vi "AutoDrawPaths.vi"(1 "RoutineName":string="untitled", 2 "Background File Path":path, 3 "RoutineSteps":T2[](array[typedef]) {"ArmPath"."ExtendTrajectory"."Time (ms)" items=["TrajectoryDuration_0ms"=0, "TrajectoryDuration_5ms"=5, "TrajectoryDuration_10ms"=10, "TrajectoryDuration_20ms"=20, "TrajectoryDuration_30ms"=30, "TrajectoryDuration_40ms"=40, "TrajectoryDuration_50ms"=50, "TrajectoryDuration_100ms"=100]; "ArmPath"."RotateTrajectory"."Time (ms)" items=["TrajectoryDuration_0ms"=0, "TrajectoryDuration_5ms"=5, "TrajectoryDuration_10ms"=10, "TrajectoryDuration_20ms"=20, "TrajectoryDuration_30ms"=30, "TrajectoryDuration_40ms"=40, "TrajectoryDuration_50ms"=50, "TrajectoryDuration_100ms"=100]}) -> ()   [LabVIEW 2018]
uses:
  TypeDef/AutoPreProcessedStep.ctl
  PathPlannerSupport/TypeDefs/DrivePlanResponse.ctl
  Pathfinder/Pathfinder-LabVIEW/Pathfinder-Lib/VIs/Segment.ctl
  Implements/Arm/TypeDefs/ArmPlanResponse.ctl
  General/MotionProfiling/TypeDefs/TrajectoryPoint.ctl
  <vilib>/Rock Robotics/WPI/ThirdParty/Phoenix-LabVIEW/Motor Controller/Controls/CTRE_Phoenix_MotorControl_TrajectoryPointTimeDur.ctl
  TypeDef/AutoWaypointType.ctl
  Implements/Arm/TypeDefs/ArmTargetPosition.ctl
  Implements/TypeDefs/IntakeState.ctl
  7e158850-ddb7-454d-ad08-8f74a83b50bd.vi
  ArgosLib/ArgosLib.lvlib
  Pathfinder/Pathfinder-LabVIEW/Pathfinder-Lib/Pathfinder.lvlib
panel:
  in  "Scale Factor":u8=2
  out "Image Out":T1(plugin-control)
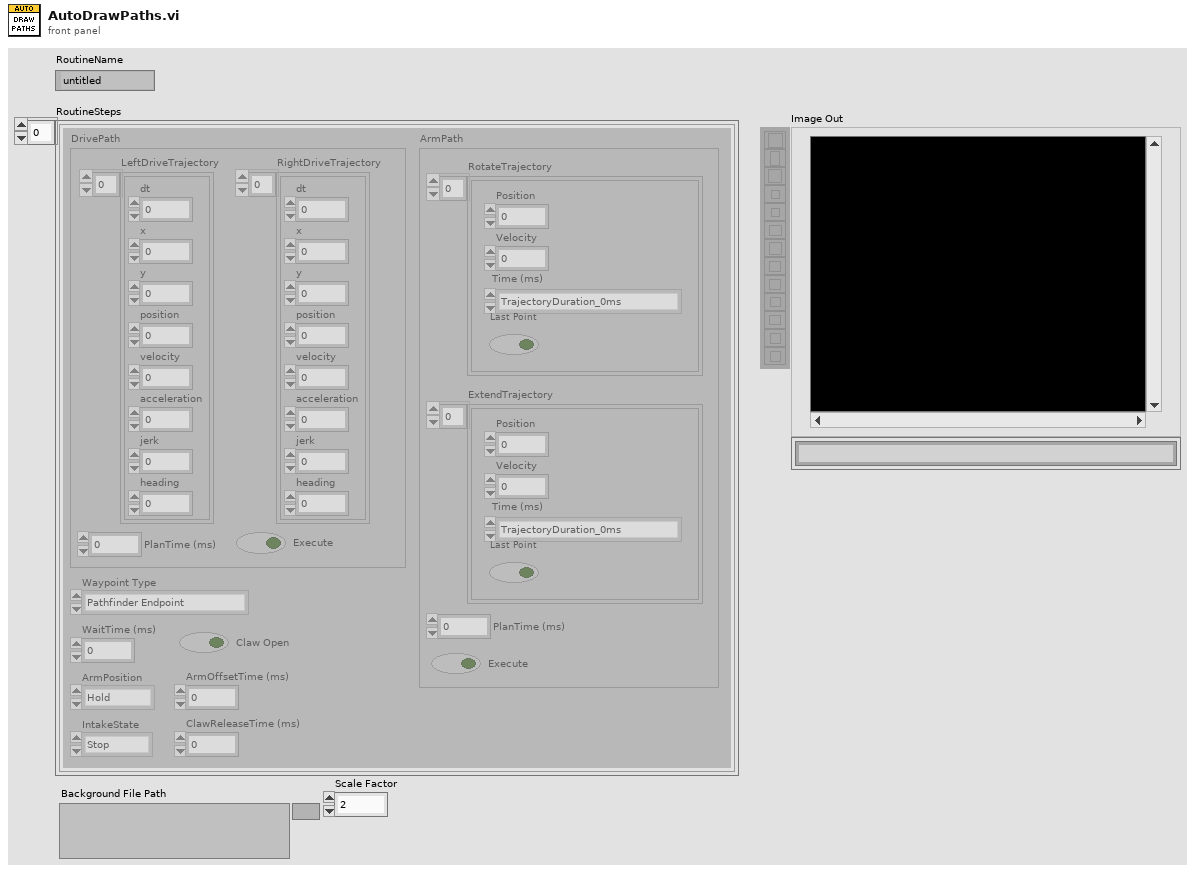
[diagram p1: front panel]
types:
  T1 = typedef "IMAQ Image.ctl" = refnum<image>
  T2 = typedef "AutoPreProcessedStep.ctl" = cluster{"DrivePath":T3, "ArmPath":T5, "Waypoint Type":T8, "WaitTime (ms)":u16, "ArmPosition":T9, "IntakeState":T10, "Claw Open":bool, "ArmOffsetTime (ms)":u16, "ClawReleaseTime (ms)":i32}
  T3 = typedef "DrivePlanResponse.ctl" = cluster{"LeftDriveTrajectory":T4[], "RightDriveTrajectory":T4[], "PlanTime (ms)":u32, "Execute":bool}
  T4 = typedef "Pathfinder.lvlib/Segment.ctl" = cluster{"dt":dbl, "x":dbl, "y":dbl, "position":dbl, "velocity":dbl, "acceleration":dbl, "jerk":dbl, "heading":dbl}
  T5 = typedef "ArmPlanResponse.ctl" = cluster{"RotateTrajectory":T6[], "ExtendTrajectory":T6[], "PlanTime (ms)":u32, "Execute":bool}
  T6 = typedef "TrajectoryPoint.ctl" = cluster{"Position ":dbl, "Velocity ":dbl, "Time (ms)":T7, "Last Point":bool}
  T7 = typedef "CTRE_Phoenix_MotorControl_TrajectoryPointTimeDur.ctl" = i32
  T8 = typedef "AutoWaypointType.ctl" = enum16{"Pathfinder Endpoint", "Pathfinder Waypoint", "Zero-Radius Turn Endpoint", "Stationary", "Vision Assist Endpoint", "Stop"}
  T9 = typedef "ArmTargetPosition.ctl" = enum16{"Hold", "Switch", "Scale Low", "Scale High", "Climb", "Back Place"}
  T10 = typedef "IntakeState.ctl" = enum16{"Stop", "Forward", "Reverse", "Forward Open"}
  T11 = typedef "Image Type" = u32
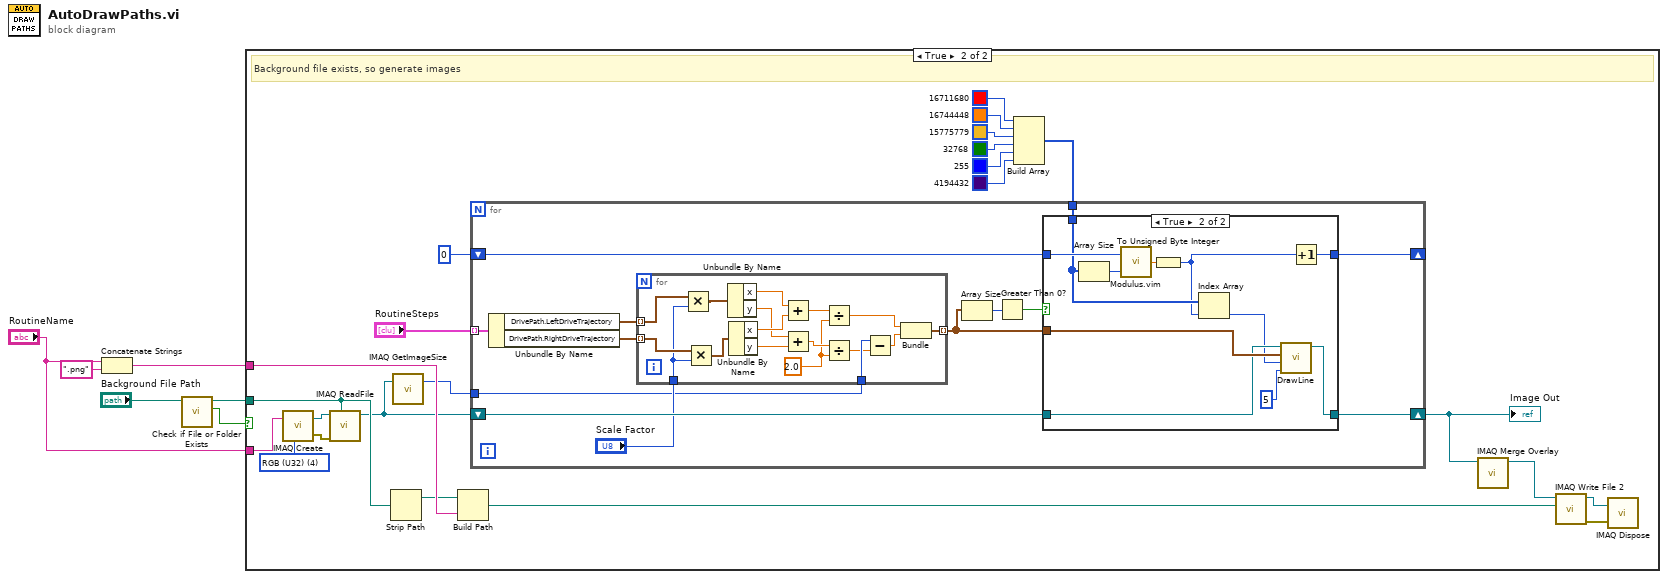
[diagram p0: block diagram]
diagram:
  n1 = Concatenate Strings("RoutineName", ".png" ("string")) -> (w5:string)
  n2 = call <vilib>:"Check if File or Folder Exists.vi"("path"="Background File Path") -> ("file or folder exists?"=w1:bool, "dup path"=w2:path)  [unwired: 8 in, 1 out]
  n3 = case shown="True" w1 {
    tunnel: w5 -> [_ w29]
    tunnel: "RoutineName" -> [_ w13]
    tunnel: w2 -> [_ w9]
    frame False {
      # "Do not generate path images"
    }
    frame True {
      w11 = T11 4 items=["Grayscale (U8)", "Grayscale (I16)", "Grayscale (SGL)", "Complex (CSG)", "RGB (U32)", "HSL (U32)", "RGB (U64)", "Grayscale (U16)"] ("Image Type")
      # "Background file exists, so generate images"
      n4 = call "IMAQ Create"("Image Name"=w13, "Image Type"=w11) -> ("New Image"=w14:T1, "error out"=w12:errorcluster)  [unwired: 3 in]
      n5 = call "IMAQ ReadFile"("File Path"=w9, "error in (no error)"=w12, "Image"=w14) -> ("Image Out"=w8:T1)  [unwired: 4 in, 4 out]
      n6 = Strip Path(path=w9) -> (stripped path=w10:path)  [unwired: 1 out]
      n7 = call "IMAQ GetImageSize"("Image"=w8) -> ("Y Resolution"=w7:i32)  [unwired: 3 in, 2 out]
      n8 = Build Path(base path=w10, name or relative path=w29) -> (appended path=w28:path)
      n9 = Build Array(u32 16711680 ("Color"), u32 16744448 ("Color"), u32 15775779 ("Color"), u32 32768 ("Color"), u32 255 ("Color"), u32 4194432 ("Color")) -> (w17:u32[])
      n10 = for {
        tunnel: "RoutineSteps" -> [w42] mode=indexing
        shift-right: [w34] -> _
        shift-left: u8 0 -> [w35]
        tunnel: w17 -> [w33]
        shift-right: [w36] -> w16
        shift-left: w8 -> [w32]
        tunnel: w7 -> [w30]
        n11 = Unbundle By Name(w42) -> ("DrivePath.LeftDriveTrajectory"=w41:T4[], "DrivePath.RightDriveTrajectory"=w40:T4[])
        n12 = for {
          tunnel: w41 -> [w58] mode=indexing
          tunnel: w40 -> [w60] mode=indexing
          tunnel: [w61] -> w37 mode=indexing
          tunnel: w30 -> [w67]
          tunnel: "Scale Factor" -> [w56]
          w62 = 2.0 ("y")
          n13 = Multiply(x=w58, y=w56) -> (x*y=w57:T4)
          n14 = Multiply(x=w60, y=w56) -> (x*y=w59:T4)
          n15 = Unbundle By Name(w57) -> ("x"=w72:dbl, "y"=w70:dbl)
          n16 = Unbundle By Name(w59) -> ("x"=w71:dbl, "y"=w69:dbl)
          n17 = Add(x=w72, y=w71) -> (x+y=w68:dbl)
          n18 = Add(x=w70, y=w69) -> (x+y=w66:dbl)
          n19 = Divide(x=w68, y=w62) -> (x/y=w64:dbl)
          n20 = Divide(x=w66, y=w62) -> (x/y=w63:dbl)
          n21 = Subtract(x=w67, y=w63) -> (x-y=w65:dbl)
          n22 = Bundle(w64, w65) -> (w61:cluster{dbl, dbl})  [unwired: 1 in]
        }
        n23 = Array Size(array=w37) -> (size(s)=w39:i32)
        n24 = Greater Than 0?(x=w39) -> (x > 0?=w38:bool)
        n25 = case shown="True" w38 {
          tunnel: w37 -> [_ w55]
          tunnel: w32 -> [w44 w54]
          tunnel: [w44 w52] -> w36
          tunnel: w35 -> [w43 w50]
          tunnel: [w43 w51] -> w34
          tunnel: w33 -> [_ w47]
          frame False {
          }
          frame True {
            n26 = Array Size(array=w47) -> (size(s)=w49:i32)
            n27 = call "Modulus.vim"("y"=w49, "x"=w50) -> ("x%y"=w48:dbl)
            n28 = To Unsigned Byte Integer(number=w48) -> (unsigned 8bit integer=w46:u8)
            n29 = Index Array(array=w47, index=w46) -> (element=w45:u32)
            n30 = call "DrawLine.vi"("Line Width (px)"=u32 5 ("Width"), "Color"=w45, "Line Endpoints"=w55, "Image"=w54) -> ("Image Out"=w52:T1)  [unwired: 7 in]
            n31 = Increment(x=w46) -> (x+1=w51:u8)
          }
        }
      }
      "Image Out" <- w16
      n32 = call "IMAQ Merge Overlay"("Image Src"=w16) -> ("Image Dst Out"=w15:T1)  [unwired: 9 in, 1 out]
      n33 = call-poly "IMAQ Write File 2"("File Path"=w28, "Image"=w15) -> ("error out"=w26:errorcluster, "Image Out (duplicate)"=w27:T1)  [unwired: 8 in]
      n34 = call "IMAQ Dispose"("Image"=w27, "error in (no error)"=w26) -> ()  [unwired: 4 in, 1 out]
    }
  }
